vi "Emballage_BDD_Certificat_CHIPREG.vi"(0 "CODE BARRE":string, 11 "error in (no error)":errorcluster) -> (4 "Saved Report Path":path=path "C:/Users/ltinguely/Desktop/test model certificat calibration CHIPREG/CHIPREG_Certif_cali__2019-02-14_083035.doc", 15 "error out":errorcluster)   [LabVIEW 2020]
uses:
  Modules/FS/60_FS_Controles/60_FS_SetGet.ctl
  controles/Clt_CertifiCal_Donnees.ctl
  controles/clt_IdentificationData.ctl
  controles/Menu_Deroulant_Gas.ctl
  controles/Menu_Deroulant_Unit.ctl
  <vilib>/Utility/NIReport.llb/Report Type.ctl
  <vilib>/Utility/NIReport.llb/NI_report.lvclass
  <vilib>/Utility/NIReport.llb/Word/NI_Word.lvclass
  <vilib>/Utility/NIReport.llb/NI_ReportGenerationCore.lvlib
panel:
  out "Temps [s] 2":dbl
  out "Temps [s]":dbl
  out "Remarque":string
  out "INDICE_PRODUIT_GPAO":i32
  out "ID_ARTICLE_GPAO":i32
  out "SN_PRODUIT_AASSIIII":i32
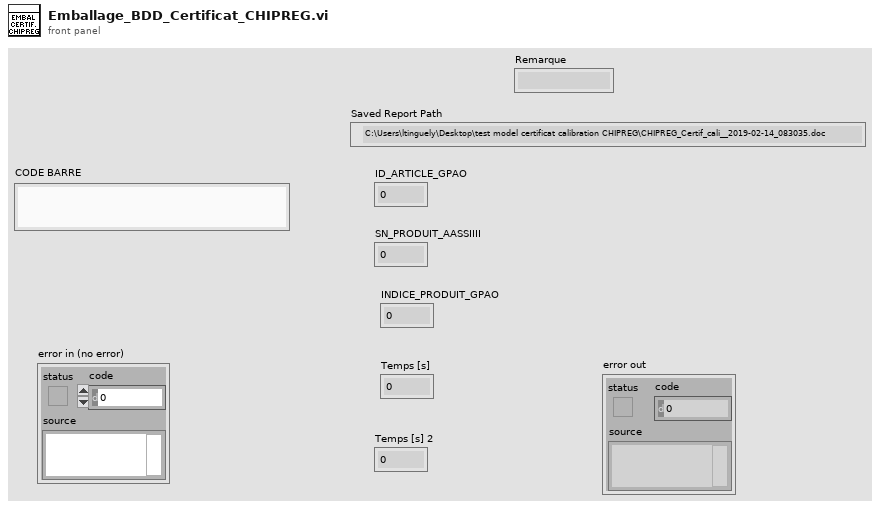
[diagram p1: front panel]
types:
  T1 = typedef "60_FS_SetGet.ctl" = enum16{"set", "get"}
  T2 = enum16{"maximized", "minimized", "normal", "no change"}
  T3 = typedef "NI_ReportGenerationCore.lvlib/Report Type.ctl" = enum16{"HTML", "Word", "Excel"}
  T4 = typedef "clt_IdentificationData.ctl" = cluster{"Part Number":string, "Suffix":string, "Description":string, "Serial Number":string, "SW Version":string, "HW Version":string, "Calibration Date (YYYYMMDDHHMMSS)":string, "Calibration Gas":T5, "calibration FullScale Interger Part":u16, "calibration FullScale Decimal Part":u16, "Device Gas":T5, "Device FullScale Interger Part":u16, "Device FullScale Decimal Part":u16, "Device Unit":T6, "Pressure Reference":u16, "Temperature Reference":u16, "Calibration Pressure":u16, "Calibration Temperature":u16, "Full Scale Accuracy":u16, "Reading Accuracy":u16}
  T5 = typedef "Menu_Deroulant_Gas.ctl" = u8
  T6 = typedef "Menu_Deroulant_Unit.ctl" = u8
  T7 = typedef "Clt_CertifiCal_Donnees.ctl" = cluster{"Fichier_xml":string, "Revision":string, "Ref_MassFlow_Sensor":string, "RefGPAO_MassFlow_Sensor":string}
  T8 = typedef "60_FS_CLT_Chemins.ctl" = cluster{"Racine_local":path, "Racine_reseau":path, "Racine_Support_Application":path, "Fichier_Journalisation":path, "Connexion_BDD_VSX":path, "Connexion_BDD_PLZ":path}
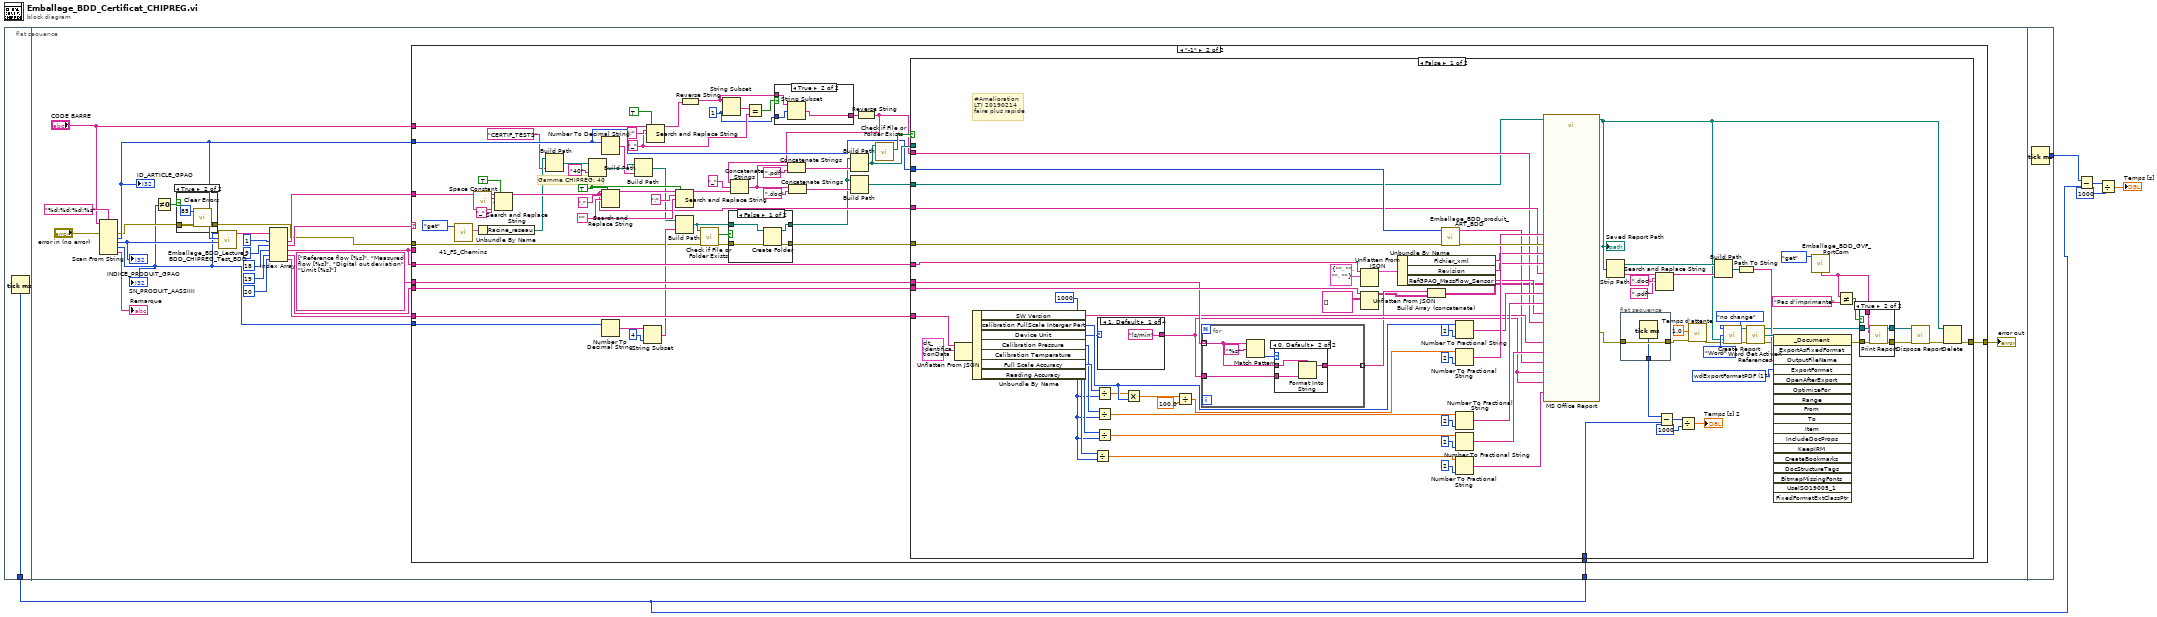
[diagram p0: block diagram]
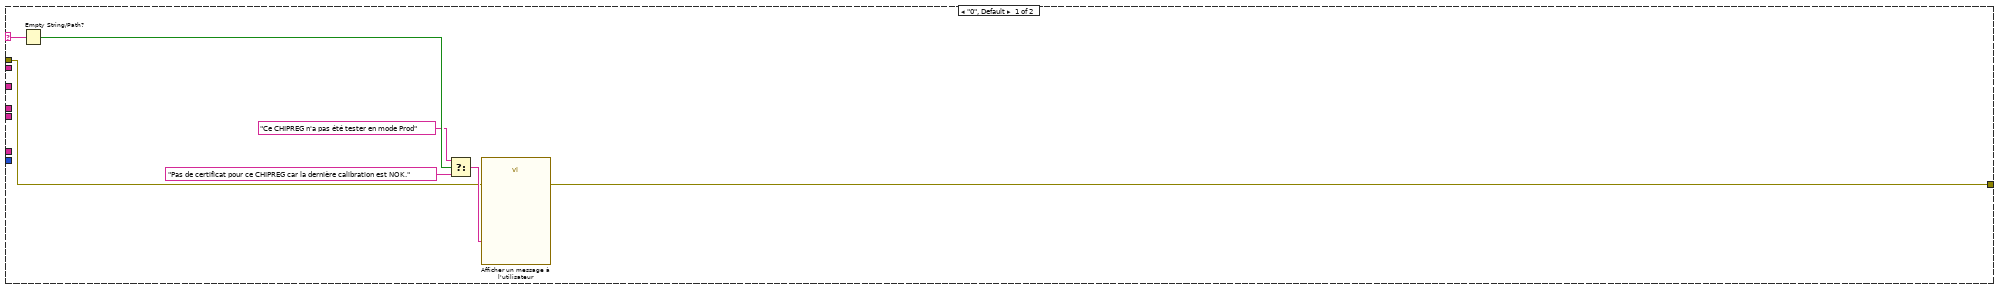
[diagram p3: hidden frame]
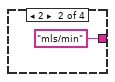
[diagram p7: hidden frame]
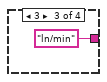
[diagram p8: hidden frame]
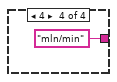
[diagram p9: hidden frame]
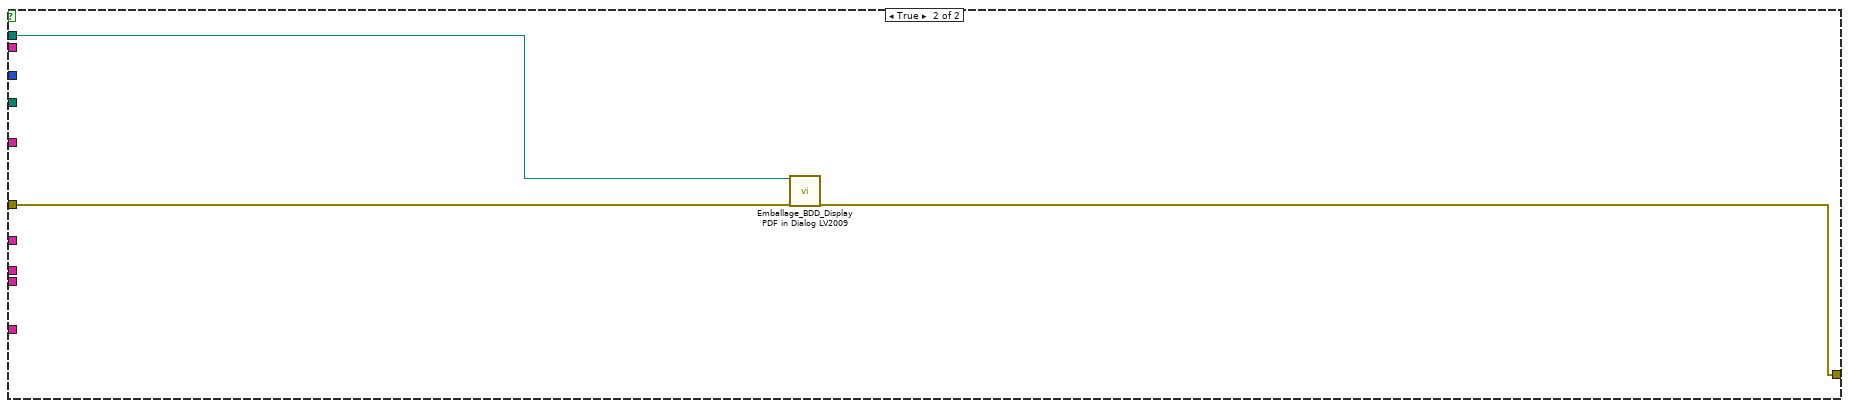
[diagram p11: hidden frame]
diagram:
  n1 = flat-sequence {
    tunnel: [w6] -> w1
    tunnel: w1 -> [w12]
    tunnel: [w216] -> w5
    frame #0 {
      n2 = Tick Count (ms)() -> (millisecond timer value=w6:u32)
    }
    frame #1 {
      n3 = Scan From String(format string="%d;%d;%d;%s" ("chaîne de format"), input string="CODE BARRE", error in="error in (no error)") -> (error out=w10:errorcluster, output 1=w14:i32, output 2=w16:i32, output 3=w7:i32, output 4=→"Remarque":string)  [unwired: 5 in, 2 out]
      "SN_PRODUIT_AASSIIII" <- w7
      "ID_ARTICLE_GPAO" <- w14
      "INDICE_PRODUIT_GPAO" <- w16
      n4 = Not Equal To 0?(x=w7) -> (x != 0?=w8:bool)
      n5 = case shown="True" w8 {
        tunnel: w10 -> [w31 w34]
        tunnel: [w31 w33] -> w9
        frame False {
        }
        frame True {
          n6 = call <vilib>:"Clear Errors.vi"("error in (no error)"=w34, "specific error code to clear (0: all)"=85) -> ("error out"=w33:errorcluster)  [unwired: 4 in, 1 out]
        }
      }
      n7 = call "Emballage_BDD_Lecture_BDD_CHIPREG_Test_BDD.vi"("INDICE_PRODUIT_GPAO"=w16, "ID_ARTICLE_GPAO"=w14, "SN_PRODUIT_AASSIIII"=w7) -> ("Donnee produit"=w18:string[])  [unwired: 7 in, 1 out]
      n8 = Index Array(array=w18, index #1=1 ("indice"), index #2=9 ("indice"), index #3=18 ("indice"), index #4=19 ("indice"), index #5=20 ("indice")) -> (element #1=w28:string, element #2=w21:string, element #3=w22:string, element #4=w24:string, element #5=w19:string)
      n9 = case shown="\"-1\"" w21 {
        selector: w21 -> [w40 _]
        tunnel: [w41 w98] -> w30
        tunnel: w28 -> [_ w91]
        tunnel: w22 -> [_ _]
        tunnel: w24 -> [_ w77]
        tunnel: string[] ["Reference flow [%s]", "Measured flow [%s]", "Digital out deviation", "Limit [%s]"] -> [_ w76]
        tunnel: w22 -> [_ w75]
        tunnel: w9 -> [w35 w56]
        tunnel: w19 -> [_ w74]
        tunnel: w14 -> [_ w66]
        tunnel: "CODE BARRE" -> [_ w73]
        tunnel: w7 -> [_ w63]
        tunnel: w12 -> [_ w50]
        frame "0", Default {
          n10 = Empty String/Path?(string/path=w40) -> (empty?=w39:bool)
          n11 = Select(t="Ce CHIPREG n'a pas été tester en mode Prod" ("cas vrai"), s=w39, f="Pas de certificat pour ce CHIPREG car la dernière calibration est NOK." ("Message")) -> (s? t:f=w37:string)
          n12 = call "Afficher un message à l'utilisateur"("error in (no error)"=w35, "Message"=w37) -> ("error out"=w41:errorcluster)  [unwired: 8 in, 1 out]
        }
        frame "-1" {
          w45 = 1 ("longueur (reste)")
          w48 = "_" ("chaîne de remplacement (\"\")")
          w86 = TRUE ("tout remplacer ? (F)")
          w92 = ""
          # "Gamme CHIPREG: 40"
          n13 = call "41_FS_Chemins.vi"("SetGet"=60_FS_SetGet."get") -> ("CLT_Chemins_out"=w69:T8)  [unwired: 9 in, 1 out]
          n14 = call <vilib>:"Space Constant.vi"() -> ("String"=w90:string)
          n15 = Unbundle By Name(w69) -> ("Racine_reseau"=w53:path)
          n16 = Search and Replace String(replace all?=TRUE ("tout remplacer ? (F)"), input string=w91, search string=w90, replace string="_" ("chaîne de remplacement (\"\")")) -> (result string=w87:string)  [unwired: 4 in, 3 out]
          n17 = Build Path(base path=w53, name or relative path="CERTIF_TESTS" ("nom ou chemin relatif")) -> (appended path=w51:path)
          n18 = Build Path(base path=w51, name or relative path="40" ("nom ou chemin relatif")) -> (appended path=w67:path)
          n19 = Number To Decimal String(number=w66) -> (decimal integer string=w65:string)  [unwired: 1 in]
          n20 = Search and Replace String(replace all?=w86, input string=w87, search string="." ("chaîne recherchée"), replace string=w92) -> (result string=w94:string)  [unwired: 4 in, 3 out]
          n21 = Number To Decimal String(number=w63) -> (decimal integer string=w62:string)  [unwired: 1 in]
          n22 = Build Path(base path=w67, name or relative path=w65) -> (appended path=w64:path)
          n23 = String Subset(string=w62, length (rest)=4 ("longueur (reste)")) -> (substring=w61:string)  [unwired: 1 in]
          n24 = Search and Replace String(replace all?=TRUE ("tout remplacer ? (F)"), input string=w73, search string=";" ("chaîne recherchée"), replace string=w48) -> (result string=w44:string)  [unwired: 4 in, 3 out]
          n25 = Search and Replace String(replace all?=w86, input string=w94, search string=":" ("chaîne recherchée"), replace string=w92) -> (result string=w88:string)  [unwired: 4 in, 3 out]
          n26 = Build Path(base path=w64, name or relative path=w61) -> (appended path=w58:path)
          n27 = Reverse String(1:w44) -> (0:w46:string)
          n28 = call <vilib>:"Check if File or Folder Exists.vi"("error in (no error)"=w56, "path"=w58) -> ("error out"=w57:errorcluster, "file or folder exists?"=w59:bool)  [unwired: 7 in, 1 out]
          n29 = String Subset(string=w46, length (rest)=w45) -> (substring=w49:string)  [unwired: 1 in]
          n30 = case shown="False" w59 {
            tunnel: w58 -> [w106 w108]
            tunnel: w57 -> [w105 w107]
            tunnel: [w104 w107] -> w55
            tunnel: [w103 w108] -> w54
            frame False {
              n31 = Create Folder(path (use dialog)=w106, error in=w105) -> (created path=w103:path, error out=w104:errorcluster)  [unwired: 1 in, 1 out]
            }
            frame True {
            }
          }
          n32 = Equal?(x=w49, y=w48) -> (x = y?=w47:bool)
          n33 = case shown="True" w47 {
            tunnel: w46 -> [w99 w102]
            tunnel: w45 -> [_ w101]
            tunnel: [w99 w100] -> w43
            frame False {
            }
            frame True {
              n34 = String Subset(string=w102, offset (0)=w101) -> (substring=w100:string)  [unwired: 1 in]
            }
          }
          n35 = Reverse String(1:w43) -> (0:w42:string)
          n36 = Concatenate Strings(w42, "_", w88) -> (w82:string)
          n37 = Concatenate Strings(w82, ".pdf" ("chaîne")) -> (w81:string)
          n38 = Concatenate Strings(w82, ".doc" ("chaîne")) -> (w83:string)
          n39 = Build Path(base path=w54, name or relative path=w81) -> (appended path=w78:path)
          n40 = Build Path(base path=w54, name or relative path=w83) -> (appended path=w97:path)
          n41 = call <vilib>:"Check if File or Folder Exists.vi"("path"=w78) -> ("file or folder exists?"=w79:bool)  [unwired: 8 in, 2 out]
          n42 = case shown="False" w79 {
            tunnel: [w145 w213] -> w98
            tunnel: w97 -> [w149 _]
            tunnel: w42 -> [w154 _]
            tunnel: w87 -> [w158 _]
            tunnel: w78 -> [_ w214]
            tunnel: w77 -> [w186 _]
            tunnel: w76 -> [w184 _]
            tunnel: w75 -> [w179 _]
            tunnel: w55 -> [w164 w215]
            tunnel: w66 -> [w162 _]
            tunnel: w74 -> [w176 _]
            tunnel: w50 -> [w126 _]
            frame False {
              w136 = 17 items=["wdExportFormatPDF"=17, "wdExportFormatXPS"=18] ("ExportFormat")
              w165 = u16 1000 ("y")
              # "#Amelioration\nLTI 20190214\nfaire plus rapide"
              n43 = Unflatten From JSON(JSON string=w176, type and defaults=T4 {"Part Number"="", "Suffix"="", "Description"="", "Serial Number"="", "SW Version"="", "HW Version"="", "Calibration Date (YYYYMMDDHHMMSS)"="", "Calibration Gas"=0, "calibration FullScale Interger Part"=0, "calibration FullScale Decimal Part"=0, "Device Gas"=0, "Device FullScale Interger Part"=0, "Device FullScale Decimal Part"=0, "Device Unit"=0, "Pressure Reference"=0, "Temperature Reference"=0, "Calibration Pressure"=0, "Calibration Temperature"=0, "Full Scale Accuracy"=0, "Reading Accuracy"=0} ("clt_IdentificationData")) -> (value=w175:T4)  [unwired: 5 in, 1 out]
              n44 = Unbundle By Name(w175) -> ("SW Version"=w153:string, "calibration FullScale Interger Part"=w174:u16, "Device Unit"=w173:T6, "Calibration Pressure"=w167:u16, "Calibration Temperature"=w172:u16, "Full Scale Accuracy"=w170:u16, "Reading Accuracy"=w169:u16)
              n45 = Divide(x=w169, y=w165) -> (x/y=w123:dbl)
              n46 = Divide(x=w170, y=w165) -> (x/y=w166:dbl)
              n47 = Divide(x=w167, y=w165) -> (x/y=w168:dbl)
              n48 = Divide(x=w172, y=w165) -> (x/y=w171:dbl)
              n49 = case shown="1, Default" w173 {
                tunnel: ["ls/min" "mls/min" "ln/min" "mln/min"] -> w150
                frame 1, Default {
                }
                frame 2 {
                }
                frame 3 {
                }
                frame 4 {
                }
              }
              n50 = Multiply(x=w166, y=w174) -> (x*y=w183:dbl)
              n51 = Divide(x=w183, y=100.0) -> (x/y=w181:dbl)
              n52 = for {
                tunnel: w184 -> [w206] mode=indexing
                tunnel: [w207] -> w147 mode=indexing
                tunnel: w150 -> [w208]
                n53 = Match Pattern(string=w206, regular expression="%s" ("expression régulière")) -> (offset past match=w204:i32)  [unwired: 1 in, 3 out]
                n54 = case shown="0, Default" w204 {
                  tunnel: w206 -> [w209 w212]
                  tunnel: w208 -> [_ w211]
                  tunnel: [w209 w210] -> w207
                  frame -1 {
                  }
                  frame 0, Default {
                    n55 = Format Into String(format string=w212, w211) -> (resulting string=w210:string)  [unwired: 2 in, 1 out]
                  }
                }
              }
              n56 = Unflatten From JSON(JSON string=w179, type and defaults=T7 {"Fichier_xml"="", "Revision"="", "Ref_MassFlow_Sensor"="", "RefGPAO_MassFlow_Sensor"=""} ("Clt_CertifiCal_Donnees")) -> (value=w180:T7)  [unwired: 5 in, 1 out]
              n57 = Unflatten From JSON(JSON string=w186, type and defaults=string[][] []) -> (value=w146:string[][])  [unwired: 5 in, 1 out]
              n58 = Unbundle By Name(w180) -> ("Fichier_xml"=w160:string, "Revision"=w159:string, "RefGPAO_MassFlow_Sensor"=w155:string)
              n59 = Build Array (concatenate)(w147, w146) -> (w148:string[][])
              n60 = call "Emballage_BDD_produit_ART_BDD.vi"("Error in"=w164, "ID_ARTICLE"=w162) -> ("Error out"=w163:errorcluster, "ART produit"=w151:string)  [unwired: 8 in]
              n61 = Number To Fractional String(number=w174, precision (6)=i16 2 ("précision (6)")) -> (F-format string=w157:string)  [unwired: 2 in]
              n62 = Number To Fractional String(number=w181, precision (6)=i16 2 ("précision (6)")) -> (F-format string=w161:string)  [unwired: 2 in]
              n63 = Number To Fractional String(number=w168, precision (6)=i16 2 ("précision (6)")) -> (F-format string=w156:string)  [unwired: 2 in]
              n64 = Number To Fractional String(number=w171, precision (6)=i16 2 ("précision (6)")) -> (F-format string=w152:string)  [unwired: 2 in]
              n65 = Number To Fractional String(number=w123, precision (6)=i16 2 ("précision (6)")) -> (F-format string=w122:string)  [unwired: 2 in]
              n66 = call "MS Office Report"("Path to Save Report"=w149, "AccuracyFullscale"=w161, "AccuryReading"=w122, "Calibration"=w160, "CalibrationRevision"=w159, "Date"=w158, "error in (no error)"=w163, "Doonees"=w148, "Fullscale"=w157, "InletPressure"=w156, "RefMassFlow"=w155, "SerialNo"=w154, "SWVersion"=w153, "Temperature"=w152, "Type"=w151, "UnitDebit"=w150, "UnitDebit2"=w150) -> ("Saved Report Path"=w117:path, "error out"=w130:errorcluster)  [unwired: 9 in]
              "Saved Report Path" <- w117
              n67 = Strip Path(path=w117) -> (stripped path=w143:path, name=w140:string)
              n68 = flat-sequence {
                tunnel: [w199] -> w121
                tunnel: w130 -> [w199]
                tunnel: [w198] -> w125
                frame #0 {
                  n69 = Tick Count (ms)() -> (millisecond timer value=w198:u32)
                }
              }
              n70 = Search and Replace String(input string=w140, search string=".doc" ("chaîne recherchée"), replace string=".pdf" ("chaîne de remplacement (\"\")")) -> (result string=w139:string)  [unwired: 5 in, 3 out]
              n71 = Subtract(x=w125, y=w126) -> (x-y=w129:u32)
              n72 = Divide(x=w129, y=u32 1000) -> (x/y=→"Temps [s] 2":dbl)
              n73 = call "Temps d'attente"("error in (no error)"=w121, "Delay Time (s)"=1.0) -> ("error out"=w116:errorcluster)  [unwired: 9 in]
              n74 = Build Path(base path=w143, name or relative path=w139) -> (appended path=w142:path)
              n75 = call <vilib>:"Create Report.vi"("window state (normal)"=T2."no change", "report type"=Report_Type."Word", "template (empty)"=w117, "error in (no error)"=w116) -> ("report out"=w113:refnum<class "NI_report.lvclass">, "error out"=w120:errorcluster)  [unwired: 10 in]
              n76 = Path To String(path=w142) -> (string=w141:string)
              n77 = call <vilib>:"Word Get ActiveX References.vi"("report in"=w113, "error in (no error)"=w120) -> ("report out"=w132:refnum<class "NI_report.lvclass">, "Word._Document"=w144:refnum<k7>, "error out"=w135:errorcluster)  [unwired: 7 in, 4 out]
              n78 = invoke class="_Document" method="ExportAsFixedFormat"(reference=w144, error in=w135, "OutputFileName"=w141, "ExportFormat"=w136) -> (error out=w114:errorcluster)  [unwired: 14 in, 17 out]
              n79 = call "Emballage_BDD_GVF_PortCom.vi"("Énum"=enum16{"get", "set"}."get") -> ("Imprimante Certif."=w111:string)  [unwired: 8 in, 6 out]
              n80 = Not Equal?(x=w111, y="Pas d'imprimante") -> (x != y?=w110:bool)
              n81 = case shown="True" w110 {
                tunnel: [w191 w197] -> w133
                tunnel: w132 -> [w192 w196]
                tunnel: [w192 w195] -> w131
                tunnel: w114 -> [w191 w194]
                tunnel: w111 -> [_ w193]
                frame False {
                }
                frame True {
                  n82 = call-dynamic "Print Report.vi"("report in"=w196, "printer name (default)"=w193, "error in (no error)"=w194) -> ("report out"=w195:refnum<class "NI_report.lvclass">, "error out"=w197:errorcluster)  [unwired: 11 in]
                }
              }
              n83 = call-dynamic "Dispose Report.vi"("report in"=w131, "error in (no error)"=w133) -> ("error out"=w134:errorcluster)  [unwired: 13 in]
              n84 = Delete(path (use dialog)=w117, error in=w134) -> (error out=w145:errorcluster)  [unwired: 3 in, 2 out]
            }
            frame True {
              n85 = call "Emballage_BDD_Display PDF in Dialog LV2009.vi"("PDF file"=w214, "error in (no error)"=w215) -> ("error out"=w213:errorcluster)  [unwired: 17 in]
            }
          }
        }
      }
      "error out" <- w30
    }
    frame #2 {
      n86 = Tick Count (ms)() -> (millisecond timer value=w216:u32)
    }
  }
  n87 = Subtract(x=w5, y=w1) -> (x-y=w4:u32)
  n88 = Divide(x=w4, y=u32 1000) -> (x/y=→"Temps [s]":dbl)
